vi "SIS.vi"   [LabVIEW 2018]
uses:
  <vilib>/Platform/TimedLoop/XDataNode/timing_clust.ctl
  <vilib>/Platform/TimedLoop/XDataNode/nitl_modes.ctl
  <vilib>/Platform/TimedLoop/XDataNode/wakeup.ctl
  Global Variables.vi
  <vilib>/Platform/TimedLoop/XDataNode/XDataNode.xnode
  <vilib>/Platform/TimedLoop/XDataNode/XDNodeRunTimeDep.lvlib
types:
  T1 = typedef "XDNodeRunTimeDep.lvlib/timing_clust.ctl" = cluster{"Expected End [f-1]":u64, "Actual End [f-1]":u64, "Finished Late? [f-1]":bool, "Expected End [i-1]":u64, "Actual End [i-1]":u64, "Finished Late? [i-1]":bool, "Expected Start [i]":u64, "Actual Start [i]":u64, "Expected Start [f]":u64, "Actual Start [f]":u64, "Source Name":string, "Structure Name":string, "Period":i64, "Deadline":i64, "Offset":i64, "Start":i64, "Priority":i32, "Timeout":i32, "Mode":T2, "Wakeup Reason":T3, "Error":errorcluster, "Source Type":string, "Secondary Source Type":string, "Global End Time":u64, "Global Start Time":u64, "Frame Duration":u64, "Iteration Duration":u64, "Assigned CPU":i32, "I/O Scan Engine Mode":u32}
  T2 = typedef "XDNodeRunTimeDep.lvlib/nitl_modes.ctl" = enum32{"No Change", "Process missed periods, maintain original phase", "Discard missed periods, maintain original phase", "Process missed periods, ignore original phase", "Discard missed periods, ignore original phase"}
  T3 = typedef "XDNodeRunTimeDep.lvlib/wakeup.ctl" = enum32{"Normal", "Aborted", "Asynchronous wakeup", "Timing source error", "Timed loop error", "Timeout"}
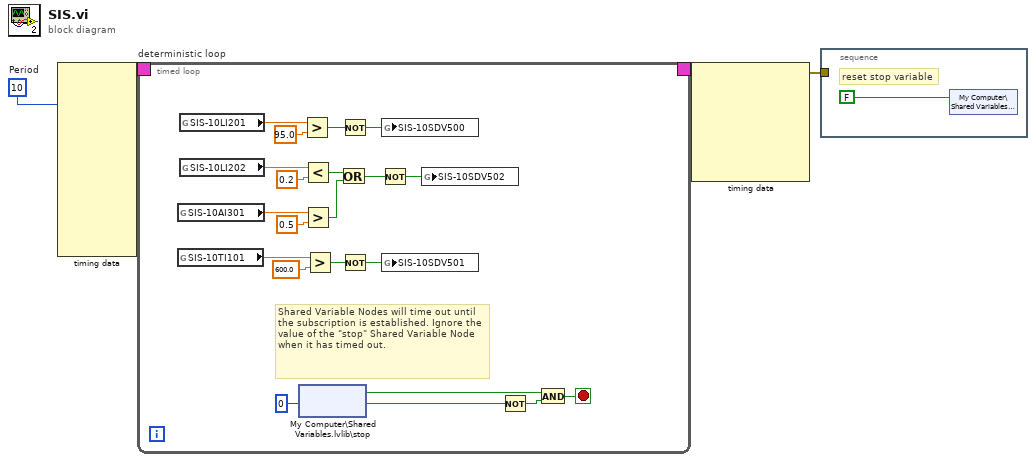
[diagram p0: block diagram]
diagram:
  w2 = i64 10  # Period
  n1 = node-c288 ("Input Node")(w2) -> (w4:T1)  [unwired: 9 in]
  n2 = timed-loop "deterministic loop" {
    timing: w4 -> [_]
    timing-out: [_] -> w3
    stop <- w25 stop-if-true
    # "Shared Variable Nodes will time out until the subscription is established. Ignore the value of the \"stop\" Shared Variable Node when it has timed out."
    n3 = global read "Global Variables.vi" "SIS-10AI301"() -> (w8:dbl)
    n4 = global read "Global Variables.vi" "SIS-10TI101"() -> (w10:dbl)
    n5 = global read "Global Variables.vi" "SIS-10LI201"() -> (w11:dbl)
    n6 = global read "Global Variables.vi" "SIS-10LI202"() -> (w9:dbl)
    n7 = shared-variable "My Computer\\Shared Variables.lvlib\\stop"(0 ("ms timeout (0)")) -> (w22:bool, w23:bool)  [unwired: 1 in, 1 out]
    n8 = Greater?(x=w11, y=95.0) -> (0:w19:bool)
    n9 = Less?(x=w9, y=0.2) -> (x < y?=w15:bool)
    n10 = Greater?(x=w8, y=0.5) -> (0:w14:bool)
    n11 = Greater?(x=w10, y=600.0) -> (0:w17:bool)
    n12 = Or(x=w15, y=w14) -> (x .or. y?=w13:bool)
    n13 = Not(x=w19) -> (.not. x?=w7:bool)
    n14 = Not(x=w17) -> (.not. x?=w6:bool)
    n15 = Not(x=w13) -> (.not. x?=w5:bool)
    n16 = global write "Global Variables.vi" "SIS-10SDV500"(w7) -> ()
    n17 = global write "Global Variables.vi" "SIS-10SDV501"(w6) -> ()
    n18 = global write "Global Variables.vi" "SIS-10SDV502"(w5) -> ()
    n19 = Not(x=w23) -> (.not. x?=w24:bool)
    n20 = And(x=w22, y=w24) -> (x .and. y?=w25:bool)
  }
  n21 = node-c288 ("Output Node")(w3) -> (w1:errorcluster)  [unwired: 5 out]
  n22 = stacked-sequence {
    tunnel: w1 -> [_]
    frame #0 {
      # "reset stop variable"
      n23 = shared-variable "My Computer\\Shared Variables.lvlib\\stop"(FALSE) -> ()  [unwired: 1 in, 1 out]
    }
  }
